vi "Hide Panel.vi"(8 "error in":errorcluster) -> (0 "error out":errorcluster)   [LabVIEW 2021, in "Main HMI.lvlib"]
doc: "Send the Hide Panel request to the Module's Main.vi.\n_____\nBased on DQMH Dev Tools: Project Template 7.1.2.1547."
uses:
  Main HMI.lvlib
  Hide Panel Argument--cluster.ctl
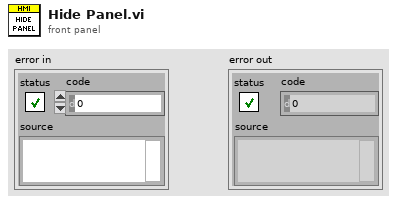
[diagram p1: front panel]
types:
  T1 = typedef "Main HMI.lvlib/Hide Panel Argument--cluster.ctl" = cluster{"Hide Panel?":bool}
  T2 = typedef "Main HMI.lvlib/Request Events--cluster.ctl" = cluster{"Stop Module":refnum<user-event>, "Show Panel":refnum<user-event>, "Hide Panel":refnum<user-event>, "Get Module Execution Status":refnum<user-event>, "Show Diagram":refnum<user-event>, "Private.Open UDP Connection":refnum<user-event>, "Private.Get UDP Info":refnum<user-event>, "Private.Recording":refnum<user-event>, "Update AIs":refnum<user-event>, "Update DOs Values":refnum<user-event>}
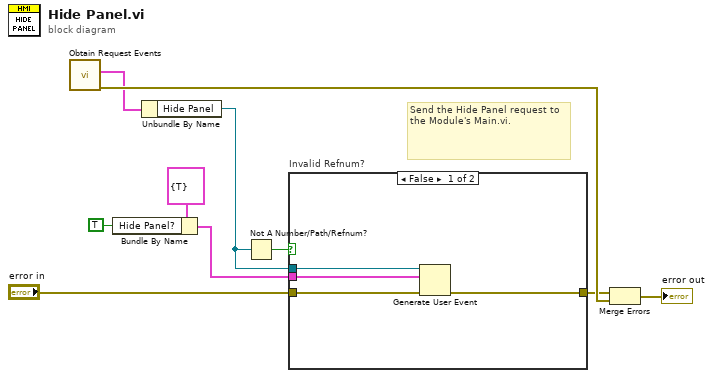
[diagram p0: block diagram]
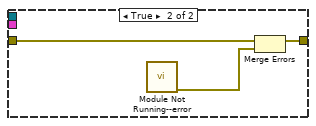
[diagram p2: hidden frame]
diagram:
  # "Send the Hide Panel request to the Module's Main.vi."
  n1 = call "Obtain Request Events.vi"() -> ("error out"=w9:errorcluster, "Main HMI Request Events"=w8:T2)  [unwired: 10 in]
  n2 = Bundle By Name(cluster=T1 {"Hide Panel?"=TRUE} ("Hide Panel Argument"), "Hide Panel?"=TRUE) -> (w2:T1)
  n3 = Unbundle By Name(w8) -> ("Hide Panel"=w6:refnum<user-event>)
  n4 = Not A Number/Path/Refnum?(number/path/refnum=w6) -> (NaN/Path/Refnum?=w7:bool)
  n5 = case "Invalid Refnum?" shown="False" w7 {
    tunnel: "error in" -> [w14 w15]
    tunnel: [w13 w16] -> w4
    tunnel: w6 -> [w12 _]
    tunnel: w2 -> [w11 _]
    frame False {
      n6 = Generate User Event(user event=w12, event data cluster=w11, error in=w14) -> (error out=w13:errorcluster)  [unwired: 1 in, 1 out]
    }
    frame True {
      n7 = call "Module Not Running--error.vi"() -> ("error out"=w17:errorcluster)  [unwired: 11 in]
      n8 = Merge Errors(w15, w17) -> (w16:errorcluster)
    }
  }
  n9 = Merge Errors(w4, w9) -> (→"error out":errorcluster)
